vi "Write motor by name.vi"(8 "error in (no error)":errorcluster, 9 "name":string, 10 "motor":refnum<class "Motor.lvclass">, 11 "ICS in":refnum<class "ICS.lvclass">) -> (0 "error out":errorcluster, 3 "ICS out":refnum<class "ICS.lvclass">)   [LabVIEW 2018, in "ICS.lvclass"]
uses:
  ICS.lvclass
  Motor/Motor.lvclass
  ICS.lvclass/ICS.ctl
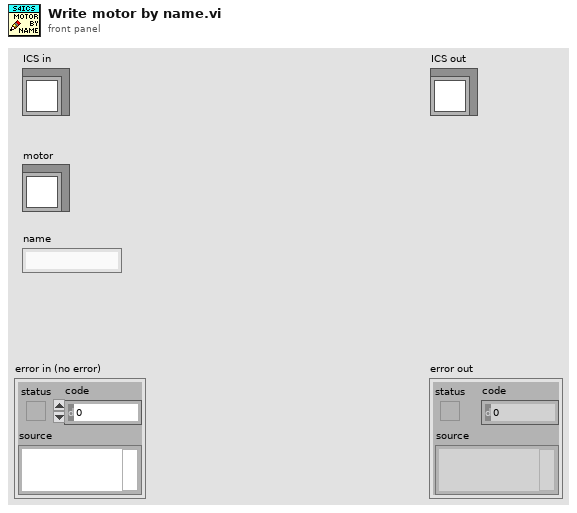
[diagram p1: front panel]
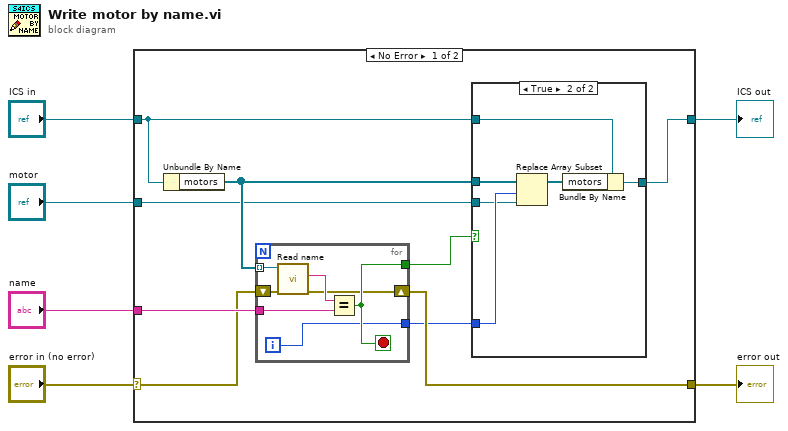
[diagram p0: block diagram]
diagram:
  n1 = case shown="No Error" "error in (no error)" {
    selector: "error in (no error)" -> [w11 w30]
    tunnel: [w10 w30] -> w5
    tunnel: [w12 w31] -> w3
    tunnel: "ICS in" -> [w13 w31]
    tunnel: "name" -> [w14 _]
    tunnel: "motor" -> [w7 _]
    frame No Error {
      n2 = Unbundle By Name(w13) -> ("motors"=w15:refnum<class "Motor.lvclass">[])
      n3 = for {
        tunnel: w15 -> [w29] mode=indexing
        tunnel: w14 -> [w27]
        tunnel: [w26] -> w9
        shift-right: [w24] -> w10
        shift-left: w11 -> [w25]
        tunnel: [w23] -> w8
        i -> [w23]
        stop <- w26 stop-if-true
        n4 = call-dynamic "Read name.vi"("error in (no error)"=w25, "Motor in"=w29) -> ("error out"=w24:errorcluster, "name"=w28:string)  [unwired: 7 in, 1 out]
        n5 = Equal?(x=w28, y=w27) -> (x = y?=w26:bool)
      }
      n6 = case shown="True" w9 {
        tunnel: w15 -> [_ w21]
        tunnel: w13 -> [w16 w20]
        tunnel: [w16 w19] -> w12
        tunnel: w8 -> [_ w18]
        tunnel: w7 -> [_ w17]
        frame False {
        }
        frame True {
          n7 = Replace Array Subset(array=w21, new element=w17, index=w18) -> (w22:refnum<class "Motor.lvclass">[])
          n8 = Bundle By Name(cluster=w20, "motors"=w22) -> (w19:refnum<class "ICS.lvclass">)
        }
      }
    }
    frame Error {
    }
  }
  "error out" <- w5
  "ICS out" <- w3
